vi "OFS_dbc_export.vi"(11 ".dbc File":path caption=".dbc File Export") -> (0 "Fehler (Ausgang)":errorcluster)   [LabVIEW 2020, in "CAN Konfig.lvlib"]
uses:
  CAN Konfig.lvlib
  Aktion FGV CAN2.ctl
  Aktion FGV CAN.ctl
  Visualisierungs Elemente/String - Ausgabefeld.ctl
  <vilib>/xnet/xnet.llb/XNET Database Create (Cluster).vi
  <vilib>/xnet/xnet.llb/XNET Database Close (Cluster).vi
  <resource>/objmgr/xnet.rc
  System Einstellungen V2/System Einstellungen V2.lvlib
  System Einstellungen V2/Aktioen FGV System.ctl
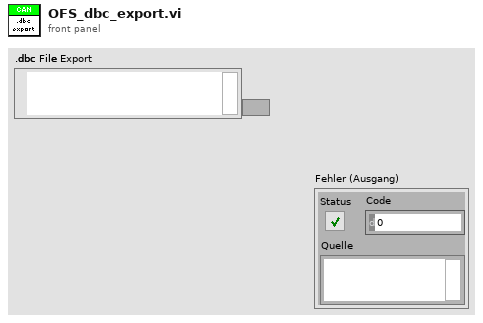
[diagram p1: front panel]
types:
  T1 = typedef "String - Ausgabefeld.ctl" = string
  T2 = enum32{"Optionsauswahl 1", "Optionsauswahl 2", "Optionsauswahl 3"}
  T3 = typedef "CAN Konfig.lvlib/Aktion FGV CAN.ctl" = enum16{"lesen", "schreiben Konfig", "Status", "Messdaten", "laden", "speichern", "CAN Data"}
  T4 = typedef "CAN Konfig.lvlib/Aktion FGV CAN2.ctl" = enum16{"lesen", "schreiben Konfig", "Status", "Messdaten", "laden", "speichern", "CAN Data", "reset more Frames avalable"}
  T5 = cluster{"OFS_NEU Database":refnum<k21>, "SAE J-1939 Database":refnum<k21>, "Status Cluster":cluster{"Status":u32[], "maxNrOfFrames":i32, "more Frames available":bool, "act. Nr of Frames":i32}}
  T6 = typedef "CAN Konfig.lvlib/CAN Messdaten.ctl" = cluster{"FTIR 1 Index":i32[], "FTIR 2 Index":i32[], "Status Index":i32[], "FT-IR Scale":sgl[], "Status Scale":sgl[], "Optionsfelder FT-IR":enum32{"Optionsauswahl 1", "Optionsauswahl 2", "Optionsauswahl 3"}, "Optionsfelder Status":enum32{"Optionsauswahl 1", "Optionsauswahl 2", "Optionsauswahl 3"}}
  T7 = typedef "CAN Konfig.lvlib/Konfig Daten PC.ctl" = cluster{"Baude Rate":T8, "COM state":u8, "Frame-ID FTIR Start":u32, "Frame-ID FTIR End":u32, "Frame-ID Status Start":u32, "Frame-ID Status End":u32, "Zustand Information":u32, "Aktion":u32, "Frame-ID FTIR Arry":u32[], "Frame-ID Status Arry":u32[], "GPS Start":u32, "Interface":refnum<k21>}
  T8 = typedef "CAN Interface.lvlib/Baude Rate.ctl" = u32
  T9 = cluster{"String":string, "Data Type":u32, "Start Bit":u32}
  T10 = typedef "System Einstellungen V2.lvlib/Aktioen FGV System.ctl" = enum16{"lesen", "laden", "speichern", "Optionen schreiben", "Zeitstempel", "Reset BMP", "Reset SQP", "Wartung", "Werkseinstellung"}
  T11 = typedef "System Einstellungen V2.lvlib/Optionen.ctl" = cluster{"Störmeldep.":bool, "Betriebszustände":bool, "AK in ppm":bool, "log Cal-Gas":bool, "log 0-Gas":bool, "Durchflusssensor 0-5V":bool, "PNS?":bool, "Mit N2 spülen":bool, "TRE08":bool, "Amium 10-Fach":bool, "Verticale Scrollbar aktiv":bool, "Loggingtakt":bool, "AK Rezeptwechsel gleich wie MKS":bool, "NG ECO":bool}
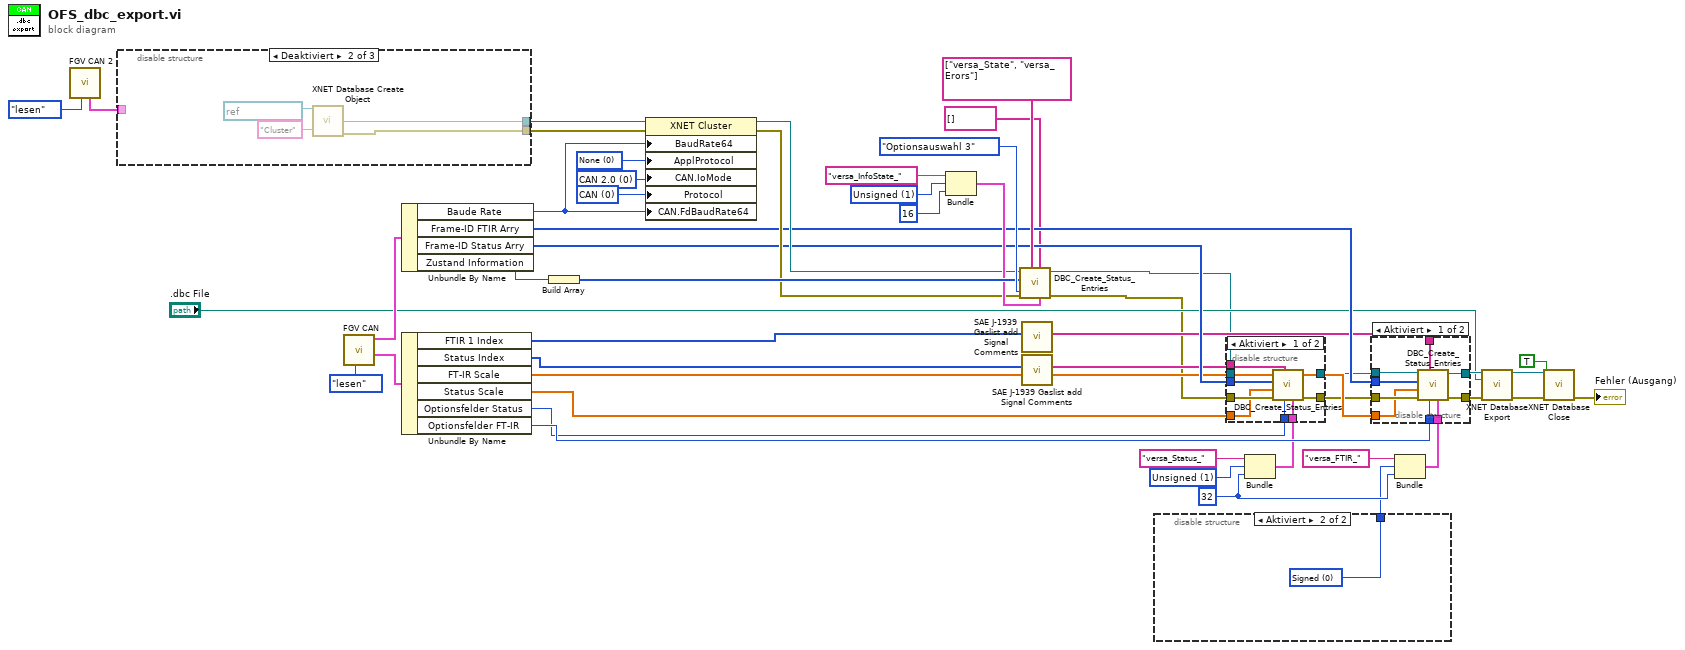
[diagram p0: block diagram]
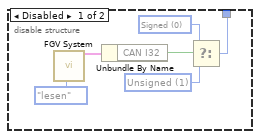
[diagram p2: hidden frame]
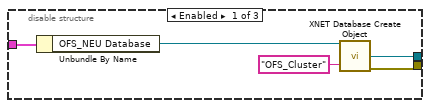
[diagram p5: hidden frame]
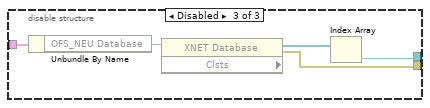
[diagram p6: hidden frame]
diagram:
  w49 = u32 32 ("Start Bit")
  w43 = u32 1 items=["Signed", "Unsigned", "IEEE Float", "Byte Array"] ("Data Type")
  w27 = u32 1 items=["Signed", "Unsigned", "IEEE Float", "Byte Array"] ("Data Type")
  w23 = u32 0 items=["CAN", "FlexRay", "LIN"] ("Protocol")
  w22 = u32 0 items=["CAN 2.0", "CAN FD", "CAN FD+BRS"] ("CAN:I/O Mode")
  w21 = u32 0 items=["None", "J1939"] ("Application Protocol")
  n1 = call "FGV CAN 2.vi"("Aktion"=Aktion_FGV_CAN2."lesen") -> ("DBC DB-Cluster"=w17:T5)  [unwired: 5 in, 5 out]
  n2 = disable-structure shown="Deaktiviert" {
    disable-tunnel: [w54 w57 w61] -> w14
    disable-tunnel: [w53 w56 w60] -> w15
    disable-tunnel: w17 -> [w52 _ w64]
    frame Enabled {
      n3 = Unbundle By Name(w52) -> ("OFS_NEU Database"=w51:refnum<k21>)
      n4 = call-poly <vilib>:"XNET Database Create Object.vi"("database in"=w51, "cluster name"="OFS_Cluster") -> ("cluster out"=w54:refnum<k21>, "error out"=w53:errorcluster)  [unwired: 11 in, 1 out]
    }
    frame Disabled {
      n5 = call-poly <vilib>:"XNET Database Create Object.vi"("database in"=refnum<k21> ":memory:", "cluster name"="Cluster") -> ("cluster out"=w57:refnum<k21>, "error out"=w56:errorcluster)  [unwired: 11 in, 1 out]
    }
    frame Disabled {
      n6 = Unbundle By Name(w64) -> ("OFS_NEU Database"=w63:refnum<k21>)
      n7 = property class="XNET Database"(reference=w63) -> (error out=w60:errorcluster, "Clsts"=w62:refnum<k21>[])  [unwired: 1 in, 1 out]
      n8 = Index Array(array=w62) -> (element=w61:refnum<k21>)  [unwired: 1 in]
    }
  }
  n9 = call "FGV CAN.vi"("Aktion"=Aktion_FGV_CAN."lesen") -> ("CAN Messdaten"=w13:T6, "Konfig Daten"=w12:T7)  [unwired: 6 in, 3 out]
  n10 = Unbundle By Name(w12) -> ("Baude Rate"=w24:T8, "Frame-ID FTIR Arry"=w37:u32[], "Frame-ID Status Arry"=w36:u32[], "Zustand Information"=w45:u32)
  n11 = Unbundle By Name(w13) -> ("FTIR 1 Index"=w8:i32[], "Status Index"=w5:i32[], "FT-IR Scale"=w33:sgl[], "Status Scale"=w16:sgl[], "Optionsfelder Status"=w38:T2, "Optionsfelder FT-IR"=w39:T2)
  n12 = Build Array(w45) -> (w46:u32[])
  n13 = property class="XNET Cluster"(reference=w14, error in=w15, "BaudRate64"=w24, "ApplProtocol"=w21, "CAN.IoMode"=w22, "Protocol"=w23, "CAN.FdBaudRate64"=w24) -> (reference out=w40:refnum<k21>, error out=w41:errorcluster)
  n14 = Bundle("String"="versa_InfoState_", "Data Type"=w43, "Start Bit"=u32 16) -> (w44:T9)  [unwired: 1 in]
  n15 = call "DBC_Create_Status_Entries.vi"("Config"=w44, "Comment"=string[] [], "Optionsfelder"=T2."Optionsauswahl 3", "Name"=T1[] ["versa_State", "versa_Erors"], "Fehler (Eingang, kein Fehler)"=w41, "Frames"=w46, "Cluster (Eingang)"=w40) -> ("Fehler (Ausgang)"=w1:errorcluster, "cluster out"=w2:refnum<k21>)  [unwired: 3 in]
  n16 = call "SAE J-1939 Gaslist add Signal Comments.vi"("FTIR 1 Index"=w8) -> ("FTIR 1 Name out"=w7:T1[])  [unwired: 10 in]
  n17 = call "SAE J-1939 Gaslist add Signal Comments.vi"("FTIR 1 Index"=w5) -> ("FTIR 1 Name out"=w4:T1[])  [unwired: 10 in]
  n18 = disable-structure shown="Aktiviert" {
    disable-tunnel: [w70 w71] -> w34
    frame Disabled {
      w68 = u32 1 items=["Signed", "Unsigned", "IEEE Float", "Byte Array"] ("Data Type")
      w69 = u32 0 items=["Signed", "Unsigned", "IEEE Float", "Byte Array"] ("Data Type")
      n19 = call "FGV System.vi"("Aktionen"=Aktioen_FGV_System."lesen") -> ("Optionen"=w66:T11)  [unwired: 12 in, 6 out]
      n20 = Unbundle By Name(w66) -> ("CAN I32"=w67:bool)
      n21 = Select(t=w69, s=w67, f=w68) -> (s? t:f=w70:u32)
    }
    frame Enabled {
      w71 = u32 0 items=["Signed", "Unsigned", "IEEE Float", "Byte Array"] ("Data Type")
    }
  }
  n22 = Bundle("String"="versa_Status_", "Data Type"=w27, "Start Bit"=w49) -> (w28:T9)  [unwired: 1 in]
  n23 = disable-structure shown="Aktiviert" {
    disable-tunnel: w36 -> [w80 _]
    disable-tunnel: w4 -> [w79 _]
    disable-tunnel: w2 -> [w72 w81]
    disable-tunnel: w1 -> [w78 w82]
    disable-tunnel: w38 -> [w77 _]
    disable-tunnel: w16 -> [w76 _]
    disable-tunnel: [w75 w82] -> w29
    disable-tunnel: [w74 w81] -> w31
    disable-tunnel: w28 -> [w73 _]
    frame Enabled {
      n24 = call "DBC_Create_Status_Entries.vi"("Config"=w73, "Optionsfelder"=w77, "Name"=w79, "Fehler (Eingang, kein Fehler)"=w78, "Scale"=w76, "Frames"=w80, "Cluster (Eingang)"=w72) -> ("Fehler (Ausgang)"=w75:errorcluster, "cluster out"=w74:refnum<k21>)  [unwired: 3 in]
    }
    frame Disabled {
    }
  }
  n25 = Bundle("String"="versa_FTIR_", "Data Type"=w34, "Start Bit"=w49) -> (w35:T9)  [unwired: 1 in]
  n26 = disable-structure shown="Aktiviert" {
    disable-tunnel: w37 -> [w91 _]
    disable-tunnel: w7 -> [w90 _]
    disable-tunnel: w31 -> [w89 w92]
    disable-tunnel: w29 -> [w88 w93]
    disable-tunnel: w39 -> [w87 _]
    disable-tunnel: w33 -> [w86 _]
    disable-tunnel: [w85 w93] -> w30
    disable-tunnel: [w84 w92] -> w32
    disable-tunnel: w35 -> [w83 _]
    frame Enabled {
      n27 = call "DBC_Create_Status_Entries.vi"("Config"=w83, "Optionsfelder"=w87, "Name"=w90, "Fehler (Eingang, kein Fehler)"=w88, "Scale"=w86, "Frames"=w91, "Cluster (Eingang)"=w89) -> ("Fehler (Ausgang)"=w85:errorcluster, "cluster out"=w84:refnum<k21>)  [unwired: 3 in]
    }
    frame Disabled {
    }
  }
  n28 = call <vilib>:"XNET Database Export.vi"("cluster in"=w32, "filepath"=".dbc File", "error in (no error)"=w30) -> ("cluster out"=w19:refnum<k21>, "error out"=w18:errorcluster)  [unwired: 11 in]
  n29 = call-poly <vilib>:"XNET Database Close.vi"("cluster in"=w19, "close all? (true)"=TRUE, "error in (no error)"=w18) -> ("error out"=→"Fehler (Ausgang)":errorcluster)  [unwired: 12 in]
